vi "Dispose.vi"(8 "error in (no error)":errorcluster, 11 "Glyph Drawer in":refnum<class "Glyph Drawer.lvclass">) -> (0 "error out":errorcluster)   [LabVIEW 2020, in "Glyph Drawer.lvlib" / "Glyph Drawer.lvclass"]
uses:
  Glyph Drawer.lvclass
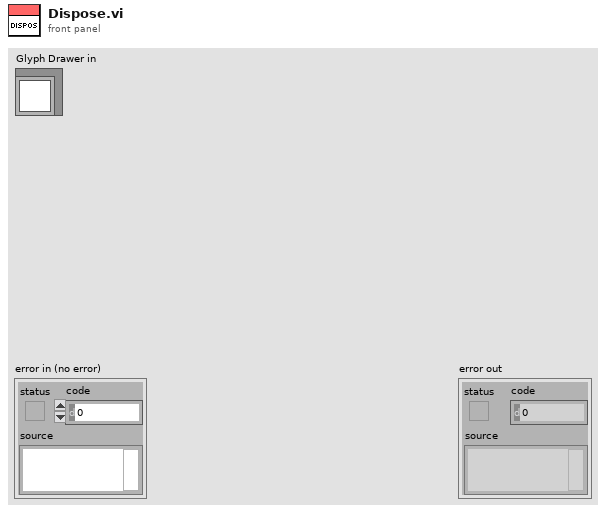
[diagram p1: front panel]
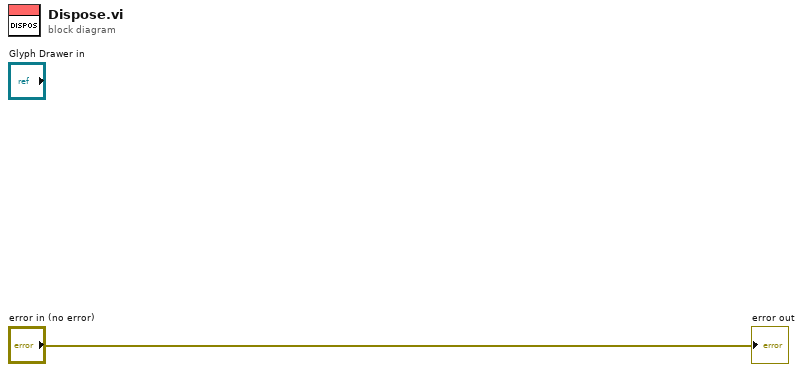
[diagram p0: block diagram]
diagram:
  "error out" <- "error in (no error)"
